vi "AnalyzeBlobs.vi"(9 "Vision Target":enum16{"Pegs", "Gears"}(ring), 10 "Blob Data":T2, 11 "Image In":T3) -> (2 "Target Data":T1, 3 "Image Out":T3)   [LabVIEW 2016]
uses:
  <vilib>/vision/Image Controls.llb/IMAQ Image.ctl
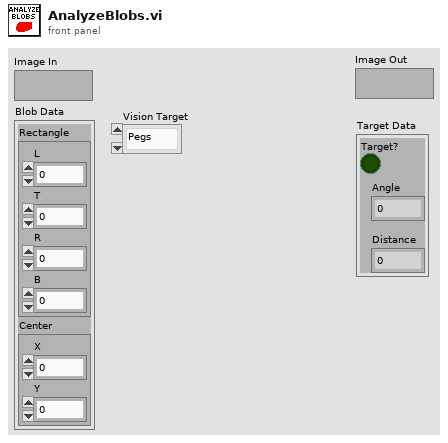
[diagram p1: front panel]
types:
  T1 = cluster{"Target?":bool, "Angle":dbl, "Distance":dbl}
  T2 = cluster{"Rectangle":cluster{"L":dbl, "T":dbl, "R":dbl, "B":dbl}, "Center":cluster{"X":dbl, "Y":dbl}}
  T3 = typedef "IMAQ Image.ctl" = refnum<image>
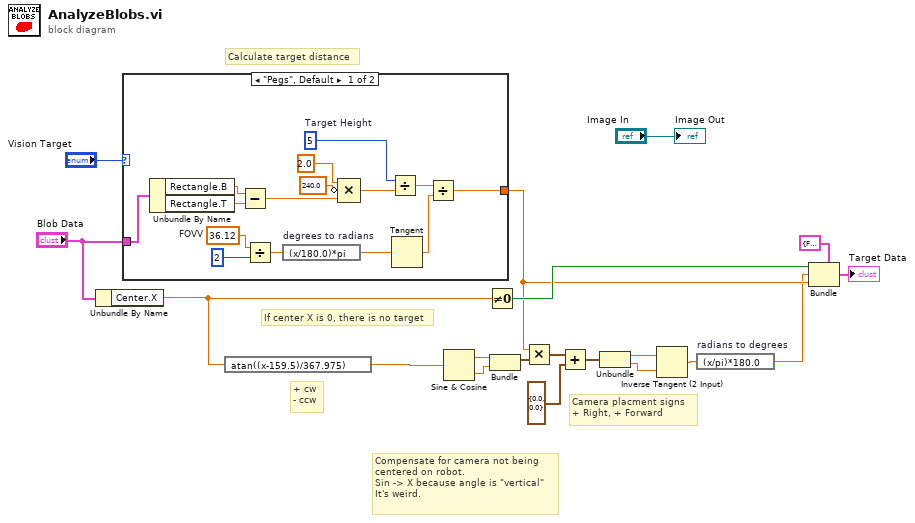
[diagram p0: block diagram]
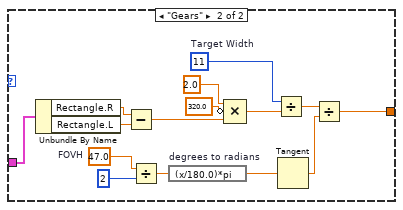
[diagram p2: hidden frame]
diagram:
  # "Camera placment signs\n+ Right, + Forward"
  # "+ cw\n- ccw"
  # "Compensate for camera not being\ncentered on robot.\nSin -> X because angle is \"vertical\"\nIt's weird."
  # "If center X is 0, there is no target"
  # "Calculate target distance"
  n1 = Unbundle By Name("Blob Data") -> ("Center.X"=w15:dbl)
  n2 = case shown="\"Pegs\", Default" "Vision Target" {
    tunnel: "Blob Data" -> [w21 w36]
    tunnel: [w20 w35] -> w10
    frame "Pegs", Default {
      w30 = 36.12  # FOVV
      w23 = 5  # Target Height
      n3 = Unbundle By Name(w21) -> ("Rectangle.B"=w28:dbl, "Rectangle.T"=w27:dbl)
      n4 = Subtract(x=w28, y=w27) -> (x-y=w29:dbl)
      n5 = Divide(x=w30, y=2) -> (x/y=w33:dbl)
      n6 = expression code="(x/180.0)*pi" "degrees to radians"(w33) -> (w34:dbl)
      n7 = Compound Arithmetic op=MULTIPLY(2.0, invert 240.0 ("value"), w29) -> (w25:dbl)
      n8 = Divide(x=w23, y=w25) -> (x/y=w32:dbl)
      n9 = Tangent(1:w34) -> (0:w22:dbl)
      n10 = Divide(x=w32, y=w22) -> (x/y=w20:dbl)
    }
    frame "Gears" {
      w45 = 47.0  # FOVH
      w38 = 11  # Target Width
      n11 = Unbundle By Name(w36) -> ("Rectangle.R"=w43:dbl, "Rectangle.L"=w42:dbl)
      n12 = Subtract(x=w43, y=w42) -> (x-y=w44:dbl)
      n13 = Divide(x=w45, y=2) -> (x/y=w48:dbl)
      n14 = expression code="(x/180.0)*pi" "degrees to radians"(w48) -> (w49:dbl)
      n15 = Compound Arithmetic op=MULTIPLY(2.0, invert 320.0 ("value"), w44) -> (w40:dbl)
      n16 = Divide(x=w38, y=w40) -> (x/y=w47:dbl)
      n17 = Tangent(1:w49) -> (0:w37:dbl)
      n18 = Divide(x=w47, y=w37) -> (x/y=w35:dbl)
    }
  }
  n19 = expression code="atan((x-159.5)/367.975)"(w15) -> (w12:dbl)
  n20 = Sine & Cosine(0:w12) -> (1:w6:dbl, 2:w5:dbl)
  n21 = Not Equal To 0?(x=w15) -> (x != 0?=w14:bool)
  n22 = Bundle(w6, w5) -> (w11:cluster{dbl, dbl})  [unwired: 1 in]
  n23 = Multiply(x=w10, y=w11) -> (x*y=w9:cluster{dbl, dbl})
  n24 = Add(x=w9, y=cluster{"X":dbl, "Y":dbl} {"X"=0.0, "Y"=0.0} ("Camera offset")) -> (x+y=w7:cluster{dbl, dbl})
  n25 = Unbundle(w7) -> (w4:dbl, w3:dbl)
  n26 = Inverse Tangent (2 Input)(1:w3, 2:w4) -> (0:w2:dbl)
  n27 = expression code="(x/pi)*180.0" "radians to degrees"(w2) -> (w1:dbl)
  n28 = Bundle(cluster=T1 {"Target?"=FALSE, "Angle"=0.0, "Distance"=0.0}, "Target?"=w14, "Angle"=w1, "Distance"=w10) -> (→"Target Data":T1)
  "Image Out" <- "Image In"
